vi "SVT Swept Sine VI Tree (DAQmx).vi"() -> ()   [LabVIEW 2017, in "SoundVib_SweptSine.lvlib"]
doc: "Shows all the user-level VIs on the Swept Sine VIs palette in a functional format. Performing swept-sine measurements requires all the VIs in the first column of this palette. Other subpalettes offer additional functionality. Swept-sine measurements developed with the NI Sound and Vibration Toolkit or the Sound and Vibration Measurement Suite follow the data-flow format depicted on the block diagram of this tree VI."
uses:
  <vilib>/addons/Sound and Vibration/svt_Swept Sine/SoundVib_SweptSine.lvlib
  <vilib>/addons/Sound and Vibration/svt_Swept Sine/SVT Initialize Swept Sine (DAQmx) (1 AO, 2 AI).vi
panel:
  in  "stop":bool
  # "SEE DIAGRAM FOR VI HIERARCHY\n\nThe diagram of this VI contains all the user-level VIs for the \nNI LabVIEW Sound and Vibration Toolset: Swept Sine Measurement."
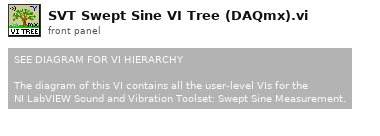
[diagram p1: front panel]
types:
  T1 = typedef "SoundVib_SweptSine.lvlib/sv_Swept Sine Task.ctl" = cluster{"source settings":cluster{"AO task name":refnum<k21>, "source":cluster{"AO physical channel":tag}[]}, "stimulus settings":cluster{"stimulus task name":refnum<k21>, "stimulus":cluster{"stimulus physical channel":tag, "channel info":T2}[]}, "response(s) settings":cluster{"response task name":refnum<k21>, "response":cluster{"response physical channel":tag, "channel info":T2}[]}, "measurement settings":cluster{"AI sampling frequency":dbl, "AO sampling frequency":dbl, "AI block size":i32, "AO block Size":i32, "block duration [ms]":dbl, "number of AI channels":i32, "device propagation delay [samples]":dbl, "total propagation time [samples]":dbl, "DUT propagation time [ms]":dbl}, "linlog":enum16{"linear", "log"}, "repeat":enum16{"off", "on"}, "frequency list":dbl[], "amplitude list":dbl[], "settling time":cluster{"settle time":dbl, "settle cycles":i32}, "integration time":cluster{"integration time":dbl, "integration cycles":i32}, "frequencies indices":cluster{"AI freq index":i32, "AO freq index":i32}, "read marks":cluster{"write index":u32, "read index":u32, "freq start index":u32, "freq stop index":u32, "# extracted":u32, "buffer type":enum16{"Invalid buffer", "Intermediate buffer", "Final buffer"}, "read/write indices":cluster{"settle time index":u32, "integration time index":u32}[], "AO index":i32, "AI index":i32, "settled":bool, "integration done":bool}, "harmonic settings":cluster{"maximum THD harmonic":u32, "harmonic mapping":u32[], "units":cluster{"THD unit":enum16{"dB", "%"}, "nth harmonic unit":enum16{"dB", "%"}, "SINAD unit":enum16{"dB", "%"}, "THD+N unit":enum16{"dB", "%"}}}, "auto resolution settings":cluster{"auto max step":i32, "slow threshold db":dbl, "fast threshold db":dbl}, "auto level settings":cluster{"auto level enable":bool, "auto level channel":u8, "ideal ref":sgl, "max level":sgl, "ref upper deviation db":sgl, "ref lower deviation db":sgl}, "offset":dbl, "ramping rate":dbl, "phase":dbl, "initialize":bool}
  T2 = typedef "svc_Channel Info.ctl" = cluster{"sensor sensitivity":dbl, "engineering units":T3, "dB reference":dbl, "custom label":string, "weighting filter":T4, "pregain":dbl}
  T3 = typedef "svc_Engineering Units Text Ring.ctl" = u16
  T4 = typedef "svc_Weighting Filter Text Ring.ctl" = u16
  T5 = typedef "SoundVib_SweptSine.lvlib/sv_Swept Sine Measurements.ctl" = cluster{"RMS stimulus":dbl[], "RMS response":dbl[], "Re [stimulus]":dbl[], "Im [stimulus]":dbl[], "Re [response]":dbl[], "Im [response]":dbl[], "THD":dbl[], "Harm[]":dbl[][], "scaled response magnitude":dbl[]}
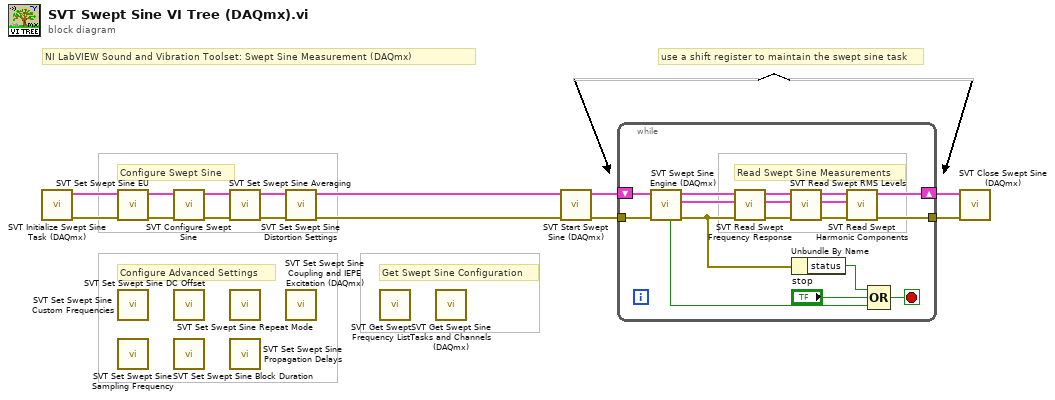
[diagram p0: block diagram]
diagram:
  # "use a shift register to maintain the swept sine task"
  # "NI LabVIEW Sound and Vibration Toolset: Swept Sine Measurement (DAQmx)"
  # "Get Swept Sine Configuration"
  # "Configure Advanced Settings"
  # "Configure Swept Sine"
  n1 = call-poly <vilib>:"SVT Initialize Swept Sine Task (DAQmx).vi"() -> ("error out"=w6:errorcluster, "swept sine task out"=w5:T1)  [unwired: 10 in]
  n2 = call <vilib>:"SVT Set Swept Sine EU.vi"("error in (no error)"=w6, "swept sine task in"=w5) -> ("error out"=w4:errorcluster, "swept sine task out"=w14:T1)  [unwired: 8 in]
  n3 = call <vilib>:"SVT Set Swept Sine Custom Frequencies.vi"() -> ()  [unwired: 10 in, 2 out]
  n4 = call <vilib>:"SVT Set Swept Sine Sampling Frequency.vi"() -> ()  [unwired: 10 in, 2 out]
  n5 = call <vilib>:"SVT Configure Swept Sine.vi"("error in (no error)"=w4, "swept sine task in"=w14) -> ("error out"=w3:errorcluster, "swept sine task out"=w13:T1)  [unwired: 8 in]
  n6 = call <vilib>:"SVT Set Swept Sine DC Offset.vi"() -> ()  [unwired: 10 in, 2 out]
  n7 = call <vilib>:"SVT Set Swept Sine Block Duration.vi"() -> ()  [unwired: 10 in, 2 out]
  n8 = call <vilib>:"SVT Set Swept Sine Averaging.vi"("error in (no error)"=w3, "swept sine task in"=w13) -> ("error out"=w2:errorcluster, "swept sine task out"=w12:T1)  [unwired: 8 in]
  n9 = call <vilib>:"SVT Set Swept Sine Repeat Mode.vi"() -> ()  [unwired: 10 in, 2 out]
  n10 = call <vilib>:"SVT Set Swept Sine Propagation Delays.vi"() -> ()  [unwired: 10 in, 2 out]
  n11 = call <vilib>:"SVT Set Swept Sine Distortion Settings.vi"("error in (no error)"=w2, "swept sine task in"=w12) -> ("error out"=w1:errorcluster, "swept sine task out"=w11:T1)  [unwired: 8 in]
  n12 = call <vilib>:"SVT Set Swept Sine Coupling and IEPE Excitation (DAQmx).vi"() -> ()  [unwired: 10 in, 2 out]
  n13 = call <vilib>:"SVT Get Swept Frequency List.vi"() -> ()  [unwired: 9 in, 3 out]
  n14 = call <vilib>:"SVT Get Swept Sine Tasks and Channels (DAQmx).vi"() -> ()  [unwired: 5 in, 7 out]
  n15 = call <vilib>:"SVT Start Swept Sine (DAQmx).vi"("error in (no error)"=w1, "swept sine task in"=w11) -> ("error out"=w9:errorcluster, "swept sine task out"=w10:T1)  [unwired: 8 in]
  n16 = while {
    shift-right: [w25] -> w7
    shift-left: w10 -> [w31]
    tunnel: w9 -> [w20]
    tunnel: [w17] -> w8
    stop <- w22 stop-if-true
    # "Read Swept Sine Measurements"
    n17 = call <vilib>:"SVT Swept Sine Engine (DAQmx).vi"("error in (no error)"=w20, "swept sine task in"=w31) -> ("error out"=w16:errorcluster, "swept sine measurements"=w30:T5, "swept sine task out"=w21:T1, "sweep done"=w23:bool)  [unwired: 4 in, 2 out]
    n18 = call <vilib>:"SVT Read Swept Frequency Response.vi"("error in (no error)"=w16, "swept sine measurements"=w30, "swept sine task in"=w21) -> ("error out"=w19:errorcluster, "dup swept sine measurements"=w29:T5, "swept sine task out"=w28:T1)  [unwired: 1 in, 5 out]
    n19 = call <vilib>:"SVT Read Swept RMS Levels.vi"("error in (no error)"=w19, "swept sine measurements"=w29, "swept sine task in"=w28) -> ("error out"=w18:errorcluster, "dup swept sine measurements"=w26:T5, "swept sine task out"=w27:T1)  [unwired: 2 in, 4 out]
    n20 = Unbundle By Name(w16) -> ("status"=w15:bool)
    n21 = call <vilib>:"SVT Read Swept Harmonic Components.vi"("error in (no error)"=w18, "swept sine measurements"=w26, "swept sine task in"=w27) -> ("error out"=w17:errorcluster, "swept sine task out"=w25:T1)  [unwired: 2 in, 5 out]
    n22 = Compound Arithmetic op=OR(w15, "stop", w23) -> (w22:bool)
  }
  n23 = call <vilib>:"SVT Close Swept Sine (DAQmx).vi"("error in (no error)"=w8, "swept sine task in"=w7) -> ()  [unwired: 9 in, 1 out]
